vi "winch down old.vi"() -> ()   [LabVIEW 2015]
uses:
  <vilib>/myRIO/Instrument Drivers/Onboard IO/PWM/typedefs/PWM Reference.ctl
  <vilib>/myRIO/Common/Instrument Driver Framework/Utilities/typedefs/myRIO Generic Hardware Reference.ctl
  <vilib>/myRIO/Common/Instrument Driver Framework/Utilities/typedefs/Hardware Version Enum.ctl
  <vilib>/myRIO/Common/Instrument Driver Framework/Utilities/typedefs/myRIO v1.0 Reference.ctl
  <vilib>/myRIO/Common/Instrument Driver Framework/Utilities/typedefs/Generic FPGA Reference.ctl
  <vilib>/myRIO/Common/Instrument Driver Framework/myRIO v1.0/PWM/typedefs/PWM Channels Enum.ctl
  <vilib>/myRIO/Instrument Drivers/Onboard IO/PWM/typedefs/PWM Configuration.ctl
  <vilib>/userdefined/High Color/nirio_resource_hc.ctl
  <vilib>/myRIO/Instrument Drivers/Onboard IO/AI/typedefs/AI Reference.ctl
  <vilib>/myRIO/Common/Instrument Driver Framework/myRIO v1.0/AI/typedefs/AI Channels List.ctl
  <vilib>/myRIO/Common/Instrument Driver Framework/myRIO v1.0/AI/typedefs/AI Channels Enum.ctl
  <vilib>/myRIO/Common/Instrument Driver Framework/Utilities/typedefs/Analog Scaling Constants List.ctl
  <vilib>/myRIO/Common/Instrument Driver Framework/Utilities/typedefs/Analog Scaling Constants.ctl
  <vilib>/myRIO/Common/Instrument Driver Framework/Utilities/vis/Is FPGA Ref Available.vi
  <vilib>/myRIO/Common/Instrument Driver Framework/myRIO v1.0/AI/vis/myRIO v1.1 Open AI.vi
  <vilib>/myRIO/Instrument Drivers/Onboard IO/AI/vis/Read.vi
  <vilib>/myRIO/Common/Instrument Driver Framework/myRIO v1.0/PWM/vis/myRIO v1.1 Open PWM.vi
  <vilib>/myRIO/Instrument Drivers/Onboard IO/PWM/vis/Set Duty Cycle and Frequency.vi
  <vilib>/myRIO/Common/Instrument Driver Framework/Utilities/vis/Validate Channels.vi
  <vilib>/myRIO/Common/Instrument Driver Framework/myRIO v1.0/AI/vis/myRIO v1.0 Reserve AI.vi
  <vilib>/myRIO/Common/Instrument Driver Framework/myRIO v1.0/PWM/vis/myRIO v1.0 Reserve PWM.vi
  <vilib>/myRIO/Common/Instrument Driver Framework/myRIO v1.0/AI/vis/myRIO v1.0 Build MUX Configuration AI.vi
  <vilib>/myRIO/Common/Instrument Driver Framework/myRIO v1.0/Resource Manager/vis/myRIO v1.0 Reserve Channel List.vi
  <vilib>/myRIO/Common/Instrument Driver Framework/myRIO v1.0/PWM/vis/myRIO v1.0 Build MUX Configuration PWM.vi
  <vilib>/myRIO/Common/Instrument Driver Framework/myRIO v1.0/Resource Manager/vis/myRIO v1.0 Reserve Channel.vi
  <vilib>/myRIO/Common/Instrument Driver Framework/myRIO v1.0/Resource Manager/vis/myRIO v1.0 Unreserve Channel.vi
  <vilib>/myRIO/Common/Instrument Driver Framework/myRIO v1.0/Resource Manager/vis/myRIO v1.0 Create Configuration List.vi
  <vilib>/myRIO/Common/Instrument Driver Framework/myRIO v1.0/Resource Manager/vis/myRIO v1.0 Build Mutex Name.vi
  <vilib>/Utility/VariantDataType/GetNumericInfo.vi
  <vilib>/Utility/error.llb/Error Cluster From Error Code.vi
  <vilib>/myRIO/Common/Instrument Driver Framework/myRIO v1.0/myRIO v1.1 Open.vi
  <vilib>/myRIO/Common/Instrument Driver Framework/Utilities/vis/IO Manager.vi
  <vilib>/myRIO/Common/Instrument Driver Framework/Utilities/vis/Configuration Manager.vi
  <vilib>/myRIO/Common/Instrument Driver Framework/myRIO v1.0/Resource Manager/vis/myRIO v1.0 Configure IO.vi
  <vilib>/myRIO/Common/Instrument Driver Framework/myRIO v1.0/myRIO v1.0 Close.vi
  <vilib>/myRIO/Common/Instrument Driver Framework/myRIO v1.0/PWM/vis/myRIO v1.0 Write PWM.vi
  <vilib>/myRIO/Common/Instrument Driver Framework/myRIO v1.0/AI/vis/myRIO v1.0 Get Scaling Constants AI.vi
  <vilib>/myRIO/Common/Instrument Driver Framework/myRIO v1.0/AI/vis/myRIO v1.0 Read AI.vi
  <vilib>/myRIO/Express VI/Onboard IO/PWM/PWM Express VI.xnode
  <vilib>/myRIO/Instrument Drivers/Onboard IO/PWM/vis/myRIO PWM Open.xnode
  <vilib>/myRIO/Express VI/Onboard IO/AI/AI Express VI.xnode
  <vilib>/myRIO/Instrument Drivers/Onboard IO/AI/vis/myRIO AI Open.xnode
  <vilib>/myRIO/Instrument Drivers/Onboard IO/PWM/PWM.lvlib
  <vilib>/myRIO/Instrument Drivers/Onboard IO/AI/AI.lvlib
panel:
  out "Stop Mining":bool
  out "position 2":dbl
  out "position 1":dbl
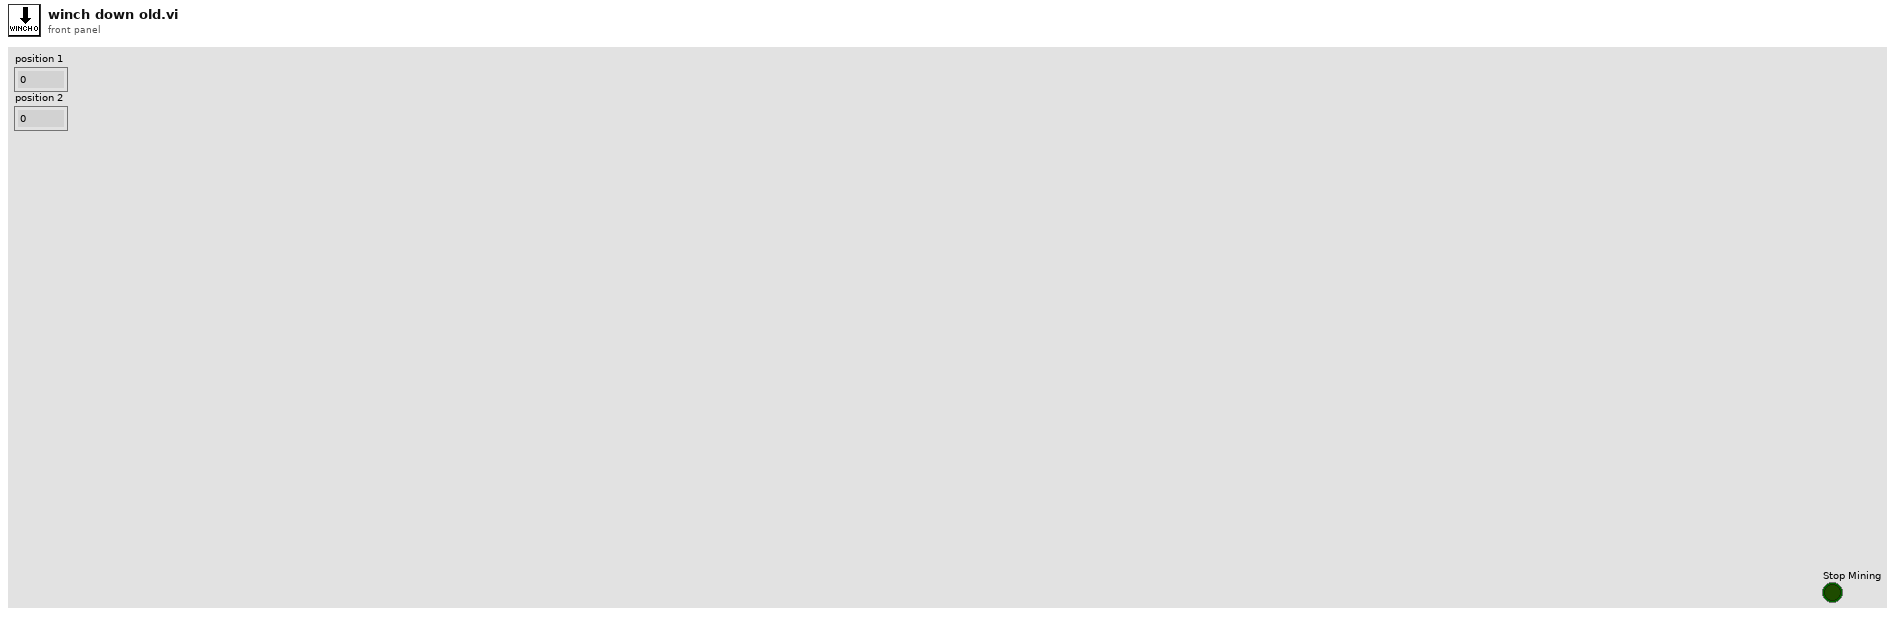
[diagram p1: front panel]
types:
  T1 = typedef "PWM.lvlib/PWM Reference.ctl" = cluster{"myRIO Reference":T2, "PWM Channels Enum":T6, "PWM Configuration":T7}
  T2 = typedef "myRIO Generic Hardware Reference.ctl" = cluster{"myRIO Model":T3, "myRIO Hardware Reference":T4}
  T3 = typedef "Hardware Version Enum.ctl" = enum16{"Unknown", "myRIO-1900", "myRIO-1950", "roboRIO"}
  T4 = typedef "myRIO v1.0 Reference.ctl" = cluster{"Generic FPGA Reference":T5, "Allow multiple opens":bool}
  T5 = typedef "Generic FPGA Reference.ctl" = refnum<k20>
  T6 = typedef "PWM Channels Enum.ctl" = enum16{"Not Connected", "C/PWM0", "C/PWM1", "A/PWM0", "A/PWM1", "A/PWM2", "B/PWM0", "B/PWM1", "B/PWM2", "PWM/PWM0", "PWM/PWM1", "PWM/PWM2", "PWM/PWM3", "PWM/PWM4", "PWM/PWM5", "PWM/PWM6", "PWM/PWM7", "PWM/PWM8", "PWM/PWM9"}
  T7 = typedef "PWM.lvlib/PWM Configuration.ctl" = cluster{"Frequency":dbl, "Duty Cycle":dbl}
  T8 = typedef "nirio_resource_hc.ctl" = tag
  T9 = typedef "AI.lvlib/AI Reference.ctl" = cluster{"myRIO Reference":T2, "AI Channels List":T10, "AI Scaling Constants List":T12}
  T10 = typedef "AI Channels List.ctl" = T11[]
  T11 = typedef "AI Channels Enum.ctl" = enum16{"Not Connected", "AudioIn/Left", "AudioIn/Right", "C/AI0", "C/AI1", "A/AI0", "A/AI1", "A/AI2", "A/AI3", "B/AI0", "B/AI1", "B/AI2", "B/AI3", "AI/AI0", "AI/AI1", "AI/AI2", "AI/AI3"}
  T12 = typedef "Analog Scaling Constants List.ctl" = T13[]
  T13 = typedef "Analog Scaling Constants.ctl" = cluster{"LSB Weight (Volts)":dbl, "Offset (Volts)":dbl, "Signed?":bool}
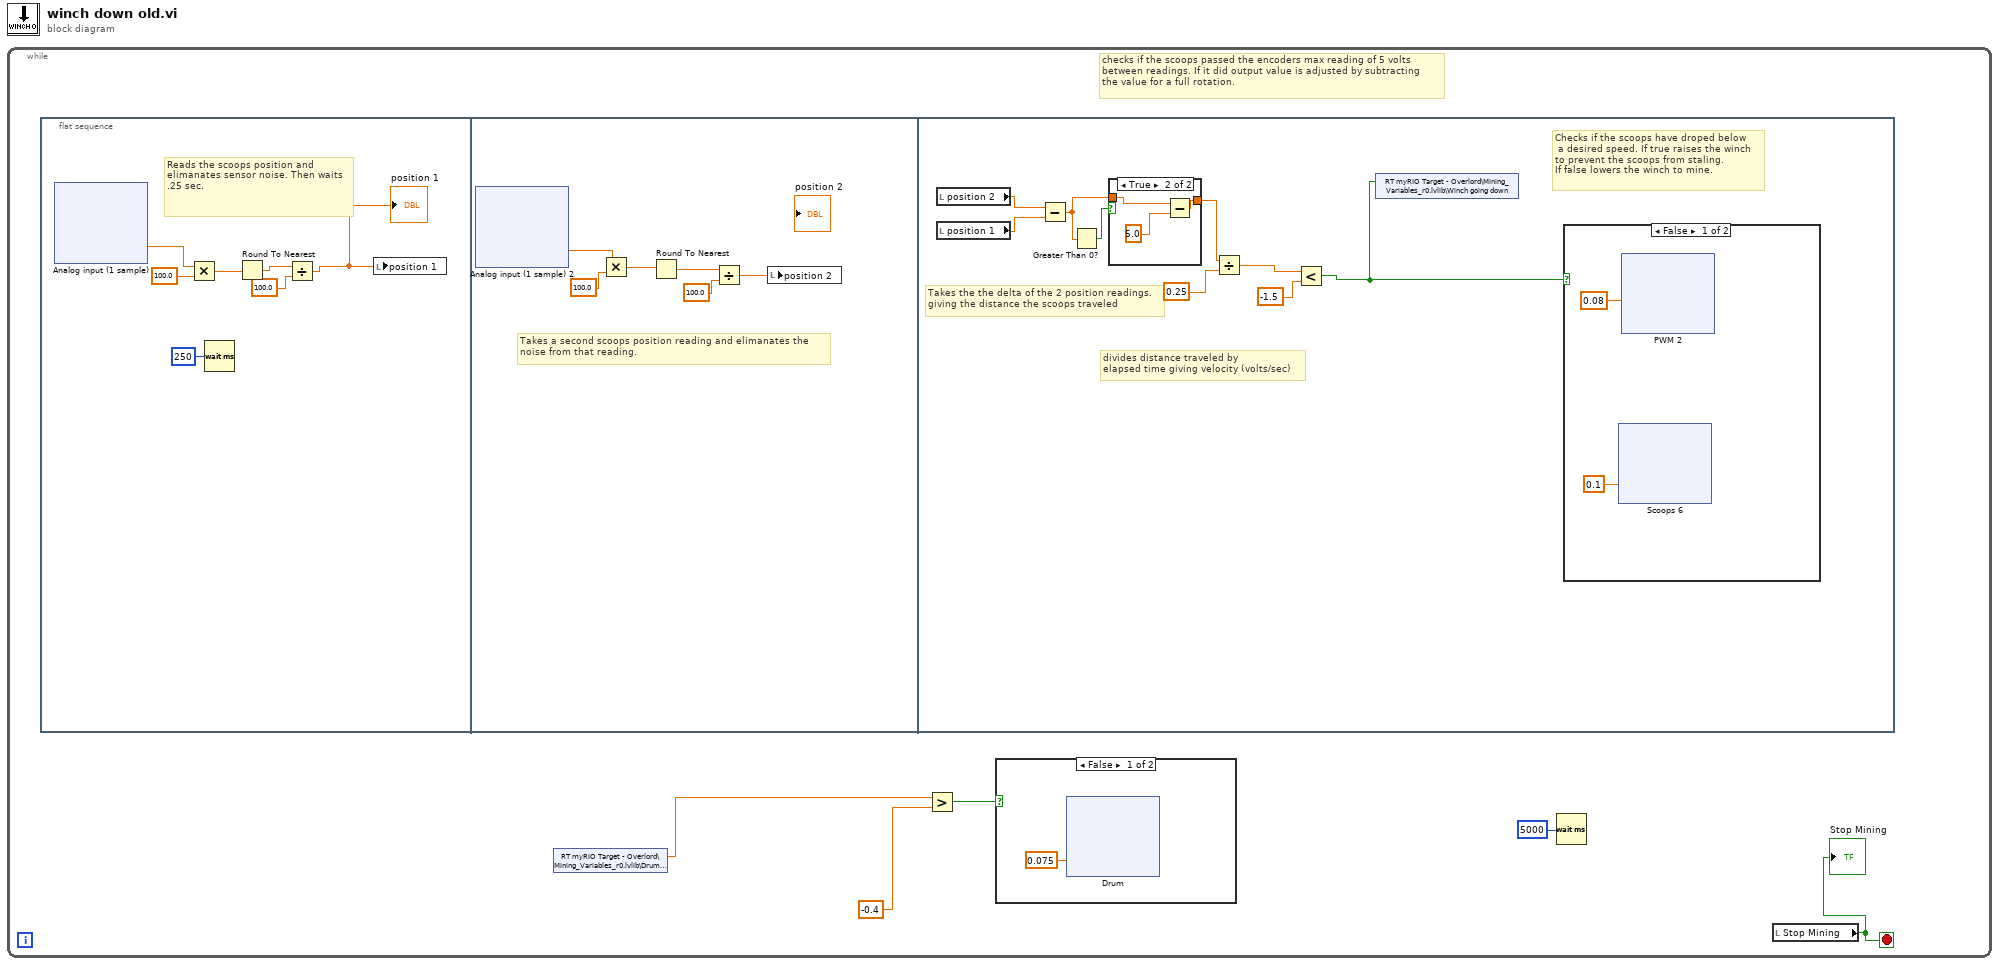
[diagram p0: block diagram]
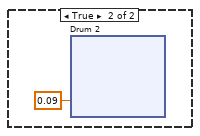
[diagram p2: hidden frame]
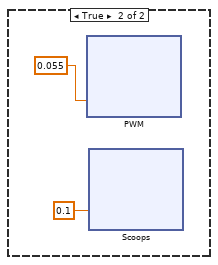
[diagram p3: hidden frame]
diagram:
  n1 = while {
    stop <- w5 stop-if-true
    # "checks if the scoops passed the encoders max reading of 5 volts\nbetween readings. If it did output value is adjusted by subtracting \nthe value for a full rotation."
    n2 = flat-sequence {
      frame #0 {
        # "Reads the scoops position and \nelimanates sensor noise. Then waits\n.25 sec."
        n3 = xnode "Analog input (1 sample)"() -> ("A/AI1 (Pin 5)"=w82:dbl)  [unwired: 1 in, 1 out]
        n4 = Multiply(x=w82, y=100.0) -> (x*y=w81:dbl)
        n5 = Wait (ms)(milliseconds to wait=u32 250) -> ()  [unwired: 1 out]
        n6 = Round To Nearest(number=w81) -> (nearest integer value=w80:dbl)
        n7 = Divide(x=w80, y=100.0) -> (x/y=w78:dbl)
        "position 1" <- w78
        n8 = local write "position 1"(w78) -> ()
      }
      frame #1 {
        # "Takes a second scoops position reading and elimanates the \nnoise from that reading."
        n9 = xnode "Analog input (1 sample) 2"() -> ("A/AI1 (Pin 5)"=w124:dbl)  [unwired: 1 in, 1 out]
        n10 = Multiply(x=w124, y=100.0) -> (x*y=w125:dbl)
        n11 = Round To Nearest(number=w125) -> (nearest integer value=w126:dbl)
        n12 = Divide(x=w126, y=100.0) -> (x/y=w127:dbl)
        n13 = local write "position 2"(w127) -> ()
      }
      frame #2 {
        # "Checks if the scoops have droped below\n a desired speed. If true raises the winch \nto prevent the scoops from staling.\nIf false lowers the winch to mine."
        # "divides distance traveled by \nelapsed time giving velocity (volts/sec)"
        # "Takes the the delta of the 2 position readings.\ngiving the distance the scoops traveled"
        n14 = local read "position 2"() -> (w173:dbl)
        n15 = local read "position 1"() -> (w172:dbl)
        n16 = Subtract(x=w173, y=w172) -> (x-y=w168:dbl)
        n17 = Greater Than 0?(x=w168) -> (x > 0?=w170:bool)
        n18 = case shown="True" w170 {
          tunnel: [w318 w321] -> w169
          tunnel: w168 -> [w318 w320]
          frame False {
          }
          frame True {
            n19 = Subtract(x=w320, y=5.0) -> (x-y=w321:dbl)
          }
        }
        n20 = Divide(x=w169, y=0.25) -> (x/y=w166:dbl)
        n21 = Less?(x=w166, y=-1.5) -> (x < y?=w165:bool)
        n22 = shared-variable "RT myRIO Target - Overlord\\Mining_Variables_r0.lvlib\\Winch going down"(w165) -> ()  [unwired: 1 in, 1 out]
        n23 = case shown="False" w165 {
          frame False {
            n24 = xnode "Scoops 6"("Duty Cycle"=0.1) -> ()  [unwired: 1 in, 1 out]
            n25 = xnode "PWM 2"("Duty Cycle"=0.08) -> ()  [unwired: 1 in, 1 out]
          }
          frame True {
            n26 = xnode "PWM"("Duty Cycle"=0.055) -> ()  [unwired: 1 in, 1 out]
            n27 = xnode "Scoops"("Duty Cycle"=0.1) -> ()  [unwired: 1 in, 1 out]
          }
        }
      }
    }
    n28 = shared-variable "RT myRIO Target - Overlord\\Mining_Variables_r0.lvlib\\Drum Accel y"() -> (w2:dbl)  [unwired: 1 in, 1 out]
    n29 = Greater?(x=w2, y=-0.4) -> (0:w4:bool)
    n30 = case shown="False" w4 {
      frame False {
        n31 = xnode "Drum"("Duty Cycle"=0.075) -> ()  [unwired: 1 in, 1 out]
      }
      frame True {
        n32 = xnode "Drum 2"("Duty Cycle"=0.09) -> ()  [unwired: 1 in, 1 out]
      }
    }
    n33 = Wait (ms)(milliseconds to wait=u32 5000) -> ()  [unwired: 1 out]
    n34 = local read "Stop Mining"() -> (w5:bool)
    "Stop Mining" <- w5
  }
